vi "MAIN.vi"() -> ()   [LabVIEW 2019]
panel:
  in  "Dec":bool
  in  "Inc":bool
  in  "Audio Device":u32 format="%.0x"
  in  "Quit":bool
  in  "Target Folder":path=path "C:/Users/tbone/Documents/GitHub/Nutella-Tsunami-Wav-Converter/convertedSamples"
  in  "Preview Sample #":i32=12
  in  "Preview":bool
  in  "Stereo":bool
  in  "Bank":i32
  in  "Convert":bool
  in  "Sample #16":path
  in  "Sample #15":path
  in  "Sample #14":path
  in  "Sample #13":path=path "C:/Users/tbone/Documents/GitHub/Nutella-Tsunami-Wav-Converter/rawSamples/CR8K/CR8KSNAR.WAV"
  in  "Sample #12":path=path "C:/Users/tbone/Documents/GitHub/Nutella-Tsunami-Wav-Converter/rawSamples/CR8K/CR8KRIM.WAV"
  in  "Sample #11":path=path "C:/Users/tbone/Documents/GitHub/Nutella-Tsunami-Wav-Converter/rawSamples/CR8K/CR8KOHAT.WAV"
  in  "Sample #10":path=path "C:/Users/tbone/Documents/GitHub/Nutella-Tsunami-Wav-Converter/rawSamples/CR8K/CR8KMCNG.WAV"
  in  "Sample #9":path=path "C:/Users/tbone/Documents/GitHub/Nutella-Tsunami-Wav-Converter/rawSamples/CR8K/CR8KLOTM.WAV"
  in  "Sample #8":path=path "C:/Users/tbone/Documents/GitHub/Nutella-Tsunami-Wav-Converter/rawSamples/CR8K/CR8KLCNG.WAV"
  in  "Sample #7":path=path "C:/Users/tbone/Documents/GitHub/Nutella-Tsunami-Wav-Converter/rawSamples/CR8K/CR8KHITM.WAV"
  in  "Sample #6":path=path "C:/Users/tbone/Documents/GitHub/Nutella-Tsunami-Wav-Converter/rawSamples/CR8K/CR8KCYMB.WAV"
  in  "Sample #5":path=path "C:/Users/tbone/Documents/GitHub/Nutella-Tsunami-Wav-Converter/rawSamples/CR8K/CR8KCOWB.WAV"
  in  "Sample #4":path=path "C:/Users/tbone/Documents/GitHub/Nutella-Tsunami-Wav-Converter/rawSamples/CR8K/CR8KCLAV.WAV"
  in  "Sample #3":path=path "C:/Users/tbone/Documents/GitHub/Nutella-Tsunami-Wav-Converter/rawSamples/CR8K/CR8KCLAP.WAV"
  in  "Sample #2":path=path "C:/Users/tbone/Documents/GitHub/Nutella-Tsunami-Wav-Converter/rawSamples/CR8K/CR8KCHAT.WAV"
  in  "Sample #1":path=path "C:/Users/tbone/Documents/GitHub/Nutella-Tsunami-Wav-Converter/rawSamples/CR8K/CR8KBASS.WAV"
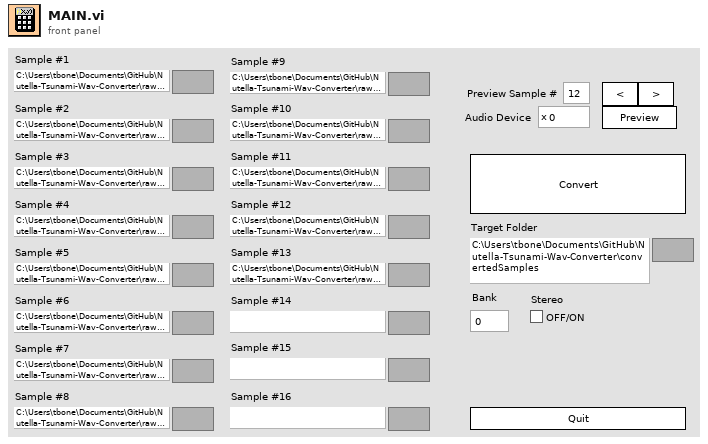
[diagram p1: front panel]
types:
  T1 = enum8{"Enabled", "Disabled", "Disabled and Grayed Out"}
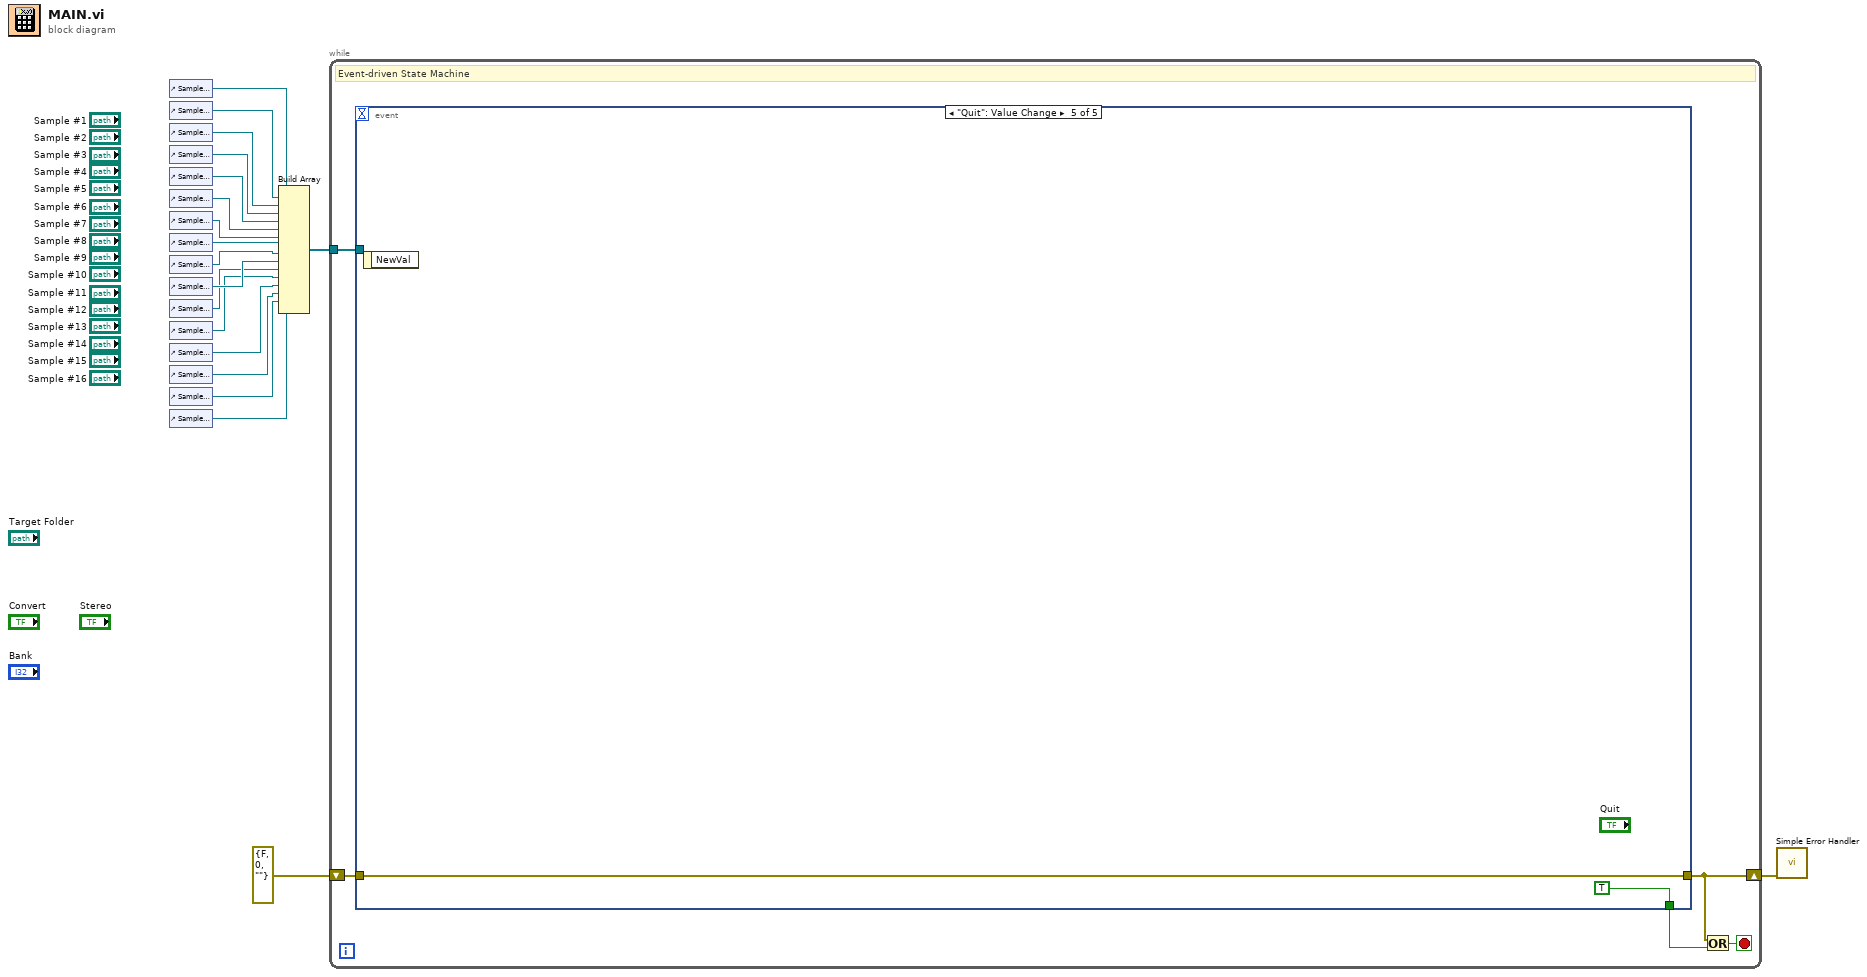
[diagram p0: block diagram]
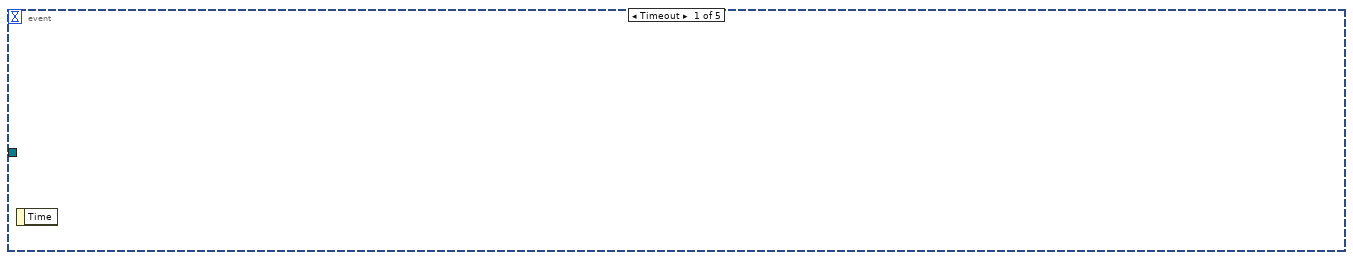
[diagram p2: hidden frame]
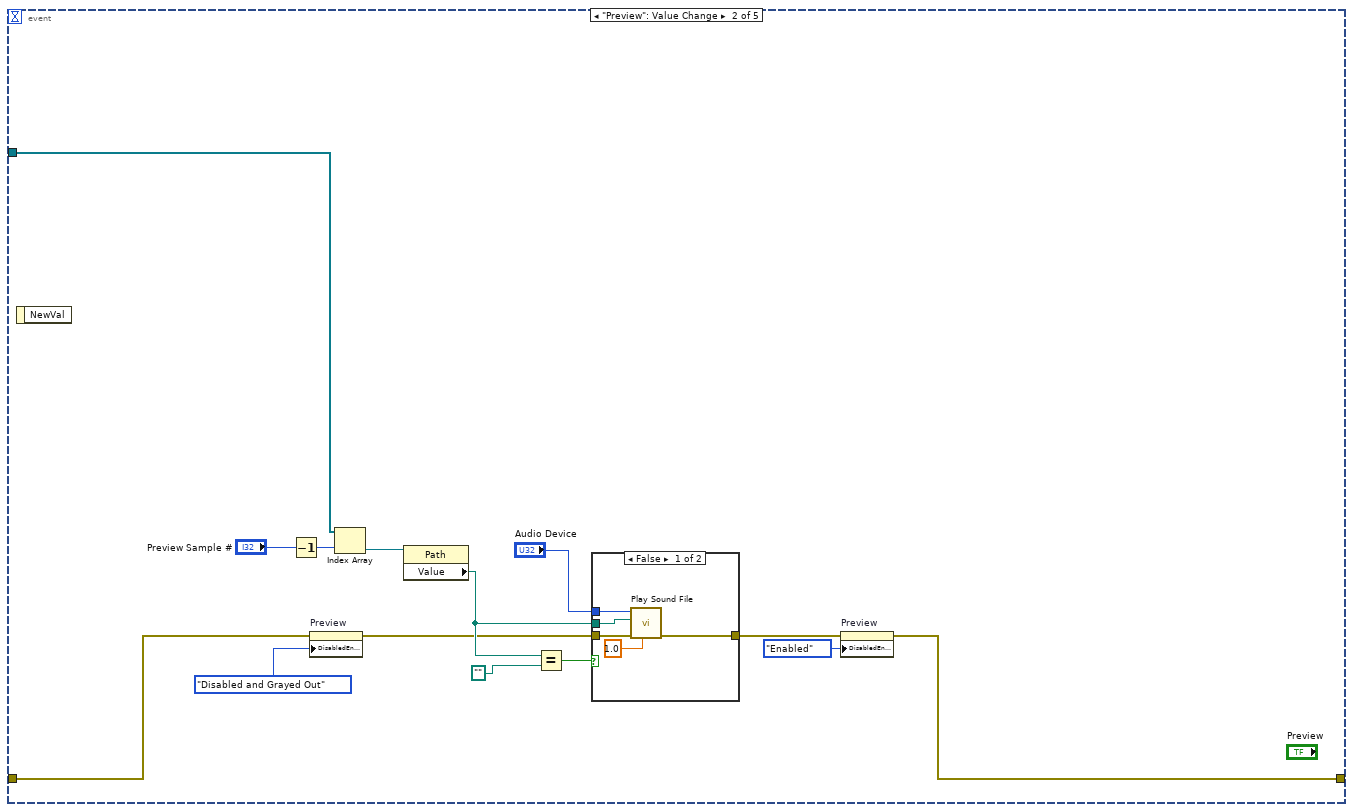
[diagram p3: hidden frame]
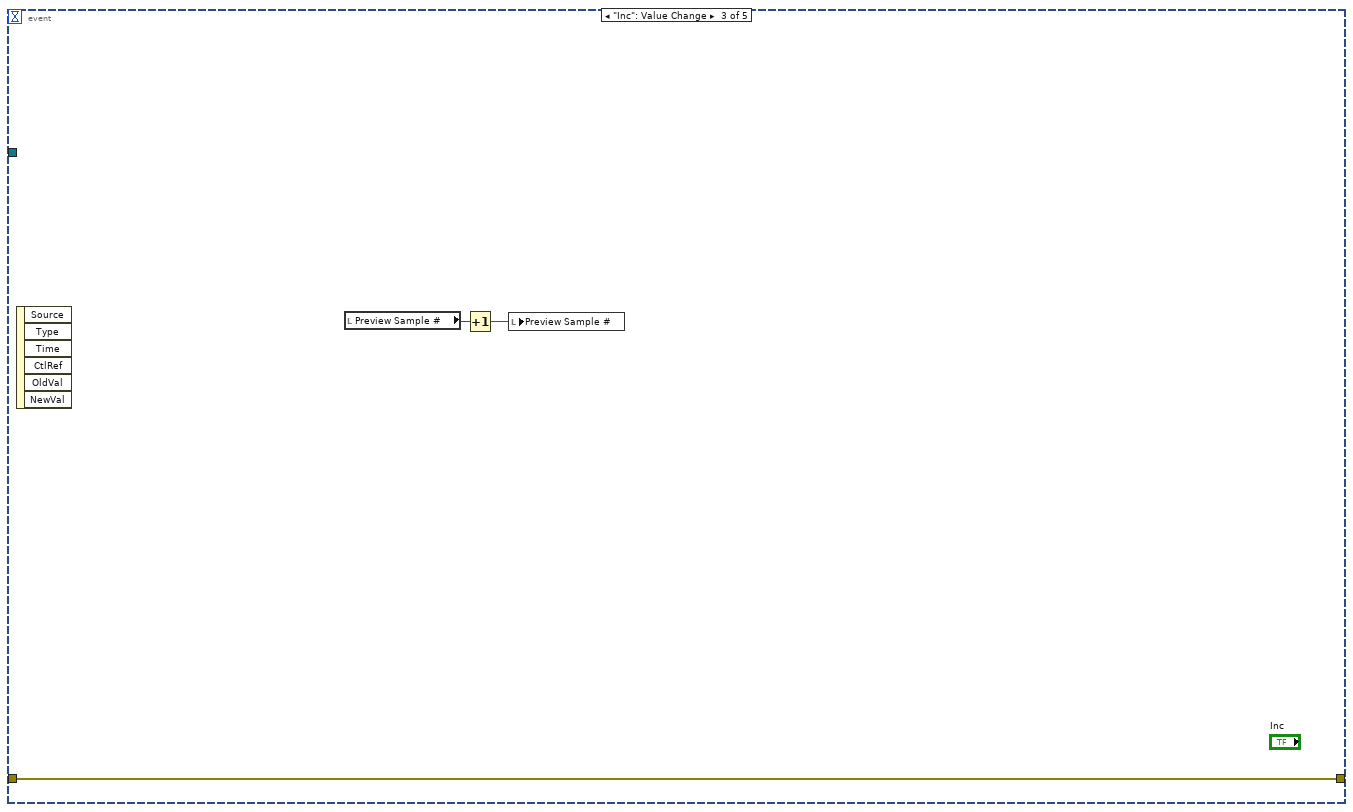
[diagram p5: hidden frame]
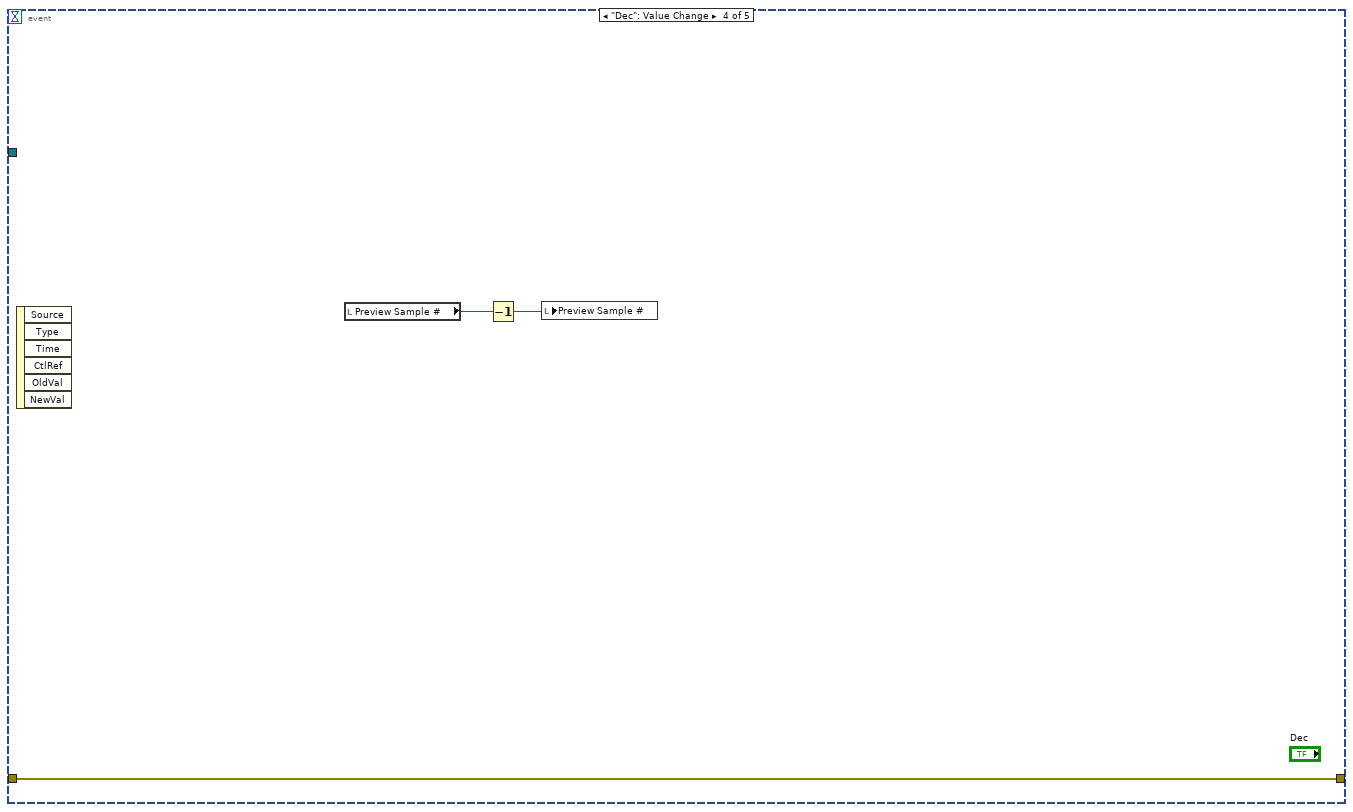
[diagram p6: hidden frame]
diagram:
  n1 = control-ref of="Sample #1"() -> (w18:refnum<vi>)
  n2 = control-ref of="Sample #2"() -> (w17:refnum<vi>)
  n3 = control-ref of="Sample #3"() -> (w16:refnum<vi>)
  n4 = control-ref of="Sample #4"() -> (w15:refnum<vi>)
  n5 = control-ref of="Sample #5"() -> (w14:refnum<vi>)
  n6 = control-ref of="Sample #6"() -> (w13:refnum<vi>)
  n7 = control-ref of="Sample #7"() -> (w12:refnum<vi>)
  n8 = control-ref of="Sample #8"() -> (w11:refnum<vi>)
  n9 = control-ref of="Sample #9"() -> (w10:refnum<vi>)
  n10 = control-ref of="Sample #10"() -> (w9:refnum<vi>)
  n11 = control-ref of="Sample #11"() -> (w8:refnum<vi>)
  n12 = control-ref of="Sample #12"() -> (w7:refnum<vi>)
  n13 = control-ref of="Sample #13"() -> (w6:refnum<vi>)
  n14 = control-ref of="Sample #14"() -> (w5:refnum<vi>)
  n15 = control-ref of="Sample #15"() -> (w4:refnum<vi>)
  n16 = control-ref of="Sample #16"() -> (w3:refnum<vi>)
  n17 = Build Array(w18, w17, w16, w15, w14, w13, w12, w11, w10, w9, w8, w7, w6, w5, w4, w3) -> (w2:refnum<vi>[])
  n18 = while {
    shift-right: [w20] -> w1
    shift-left: errorcluster {"status"=FALSE, "code"=0, "source"=""} ("error constant") -> [w24]
    tunnel: w2 -> [w23]
    stop <- w21 stop-if-true
    # "Event-driven State Machine"
    n19 = event shown="[4] \"Quit\": Value Change" {
      selector: _ -> [_ _ _ _ _]
      dyn-events: _ -> [_ _ _ _ _]
      timeout: _ -> [_ _ _ _ _]
      tunnel: [_ _ _ _ TRUE] -> w22
      tunnel: w24 -> [_ w28 w45 w50 w51]
      tunnel: [_ w26 w45 w50 w51] -> w20
      tunnel: w23 -> [_ w37 _ _ _]
      event Timeout {
        n20 = event-data() -> ()  [unwired: 1 in, 1 out]
      }
      event "Preview": Value Change {
        n21 = event-data() -> ()  [unwired: 1 in, 1 out]
        n22 = Decrement(x="Preview Sample #") -> (x-1=w31:i32)
        n23 = property on="Preview" class="Bool"(error in=w28, "DisabledEnum"=T1."Disabled and Grayed Out" ("Disabled")) -> (error out=w29:errorcluster)  [unwired: 1 in, 1 out]
        n24 = Index Array(array=w37, index=w31) -> (element=w36:refnum<vi>)
        n25 = property class="Path"(reference=w36) -> ("Value"=w33:path)  [unwired: 1 in, 2 out]
        n26 = Equal?(x=w33, y=path "") -> (x = y?=w34:bool)
        n27 = case shown="False" w34 {
          tunnel: "Audio Device" -> [w43 _]
          tunnel: w29 -> [w42 w44]
          tunnel: [w41 w44] -> w27
          tunnel: w33 -> [w40 _]
          frame False {
            n28 = call <vilib>:"Play Sound File.vi"("timeout (sec)"=1.0, "error in (no error)"=w42, "path"=w40, "device ID"=w43) -> ("error out"=w41:errorcluster)  [unwired: 6 in, 1 out]
          }
          frame True {
            # "No File"
          }
        }
        n29 = property on="Preview" class="Bool"(error in=w27, "DisabledEnum"=T1."Enabled" ("Disabled")) -> (error out=w26:errorcluster)  [unwired: 1 in, 1 out]
      }
      event "Inc": Value Change {
        n30 = event-data() -> ()  [unwired: 1 in, 6 out]
        n31 = local read "Preview Sample #"() -> (w47:i32)
        n32 = Increment(x=w47) -> (x+1=w46:i32)
        n33 = local write "Preview Sample #"(w46) -> ()
      }
      event "Dec": Value Change {
        n34 = event-data() -> ()  [unwired: 1 in, 6 out]
        n35 = local read "Preview Sample #"() -> (w49:i32)
        n36 = Decrement(x=w49) -> (x-1=w48:i32)
        n37 = local write "Preview Sample #"(w48) -> ()
      }
      event "Quit": Value Change {
        n38 = event-data() -> ()  [unwired: 1 in, 1 out]
      }
    }
    n39 = Or(x=w20, y=w22) -> (x .or. y?=w21:bool)
  }
  n40 = call <vilib>:"Simple Error Handler.vi"("error in (no error)"=w1) -> ()  [unwired: 4 in, 5 out]
